vi "TCP Multiple Connections - Server.vi"() -> ()   [LabVIEW 2016]
doc: "该范例为支持客户端VI多个连接的TCP服务器VI。"
uses:
  controls/TCP Multiple Connections State.ctl
  controls/TCP Multiple Connections Data.ctl
panel:
  out "Boolean 3":bool
  out "flag":bool
  out "old":string
  in  "Boolean 2":bool
  in  "Boolean":bool
  out "值":cluster{"数值输入控件":dbl}
  out "错误输出":errorcluster
  out "temp":dbl format="%.2f"
  in  "loop":dbl
  out "sending msg":string
  out "data out":string
  in  "停止":bool
  out "连接数":i32
  # "概述：演示使用TCP函数初始化可向多个客户端VI发送数据的TCP服务器。\n操作步骤:\n1.运行VI。\n2.打开TCP Multiple Connections - Client 1.vi并按照前面板上的说明操作。\n3.打开TCP Multiple Connections - Client 2.vi并按照前面板上的说明操作。\n4.单击停止 停止VI运行。"
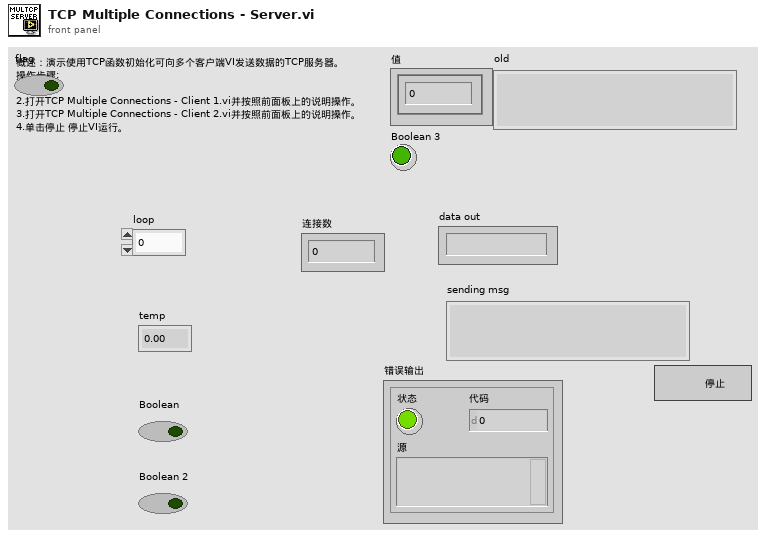
[diagram p1: front panel]
types:
  T1 = typedef "TCP Multiple Connections Data.ctl" = cluster{"客户端":refnum<k5>[], "侦听器":refnum<k5>}
  T2 = typedef "TCP Multiple Connections State.ctl" = enum16{"Initialize", "Status Check", "Send Data", "Stop"}
  T3 = enum16{"Standard", "Buffered", "CRLF", "Immediate"}
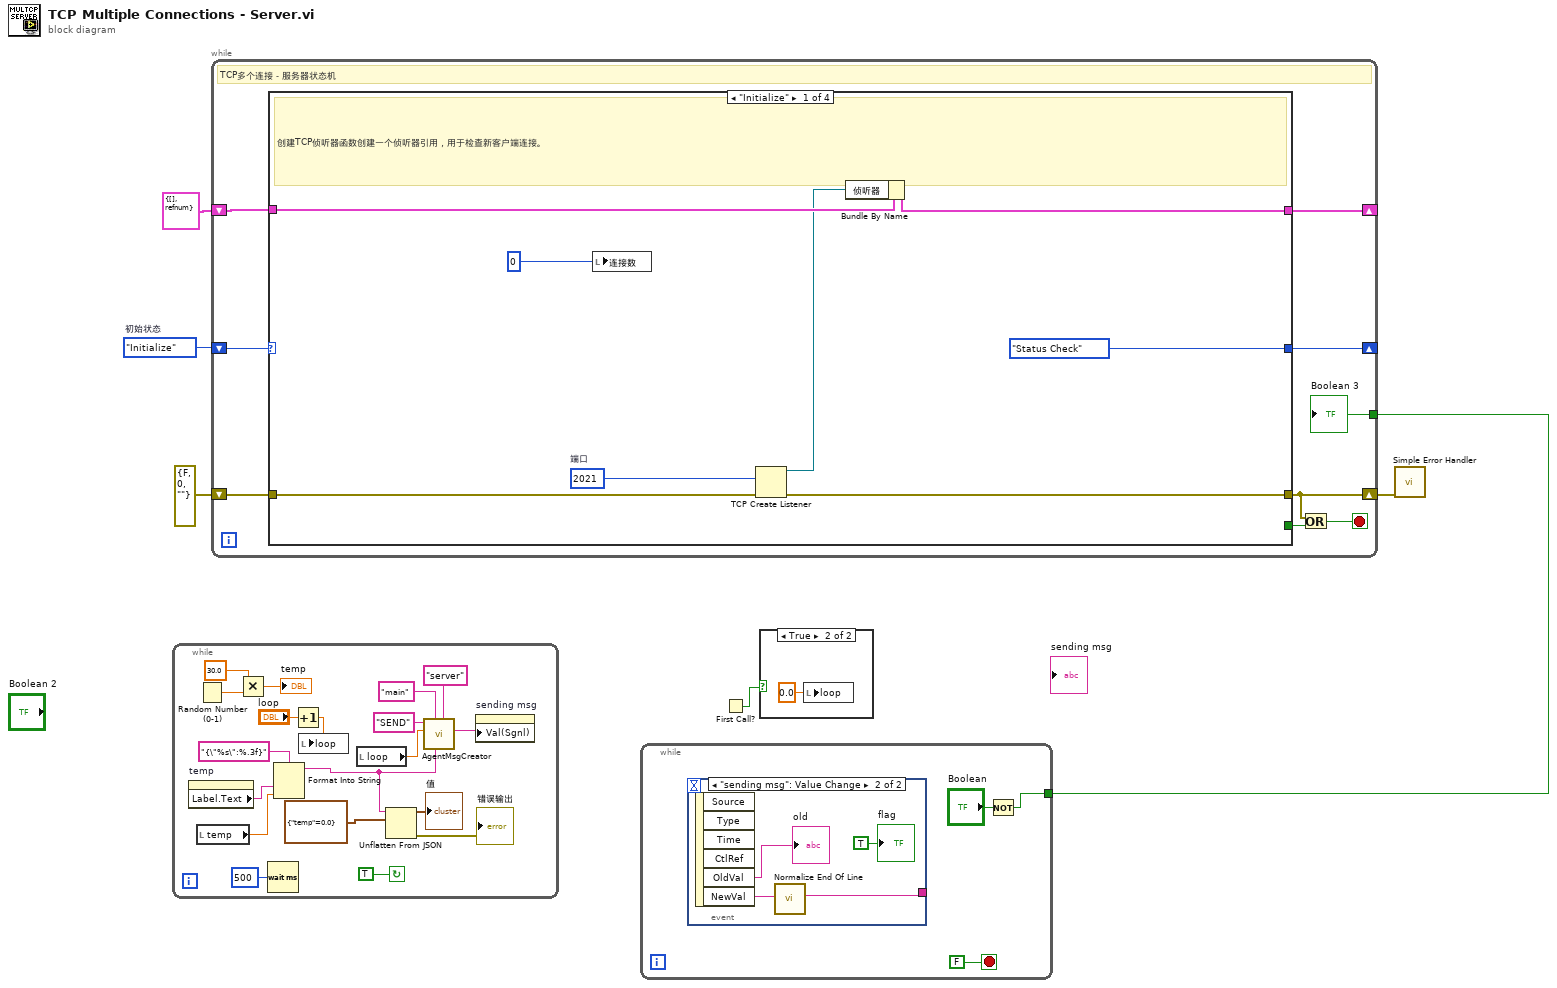
[diagram p0: block diagram]
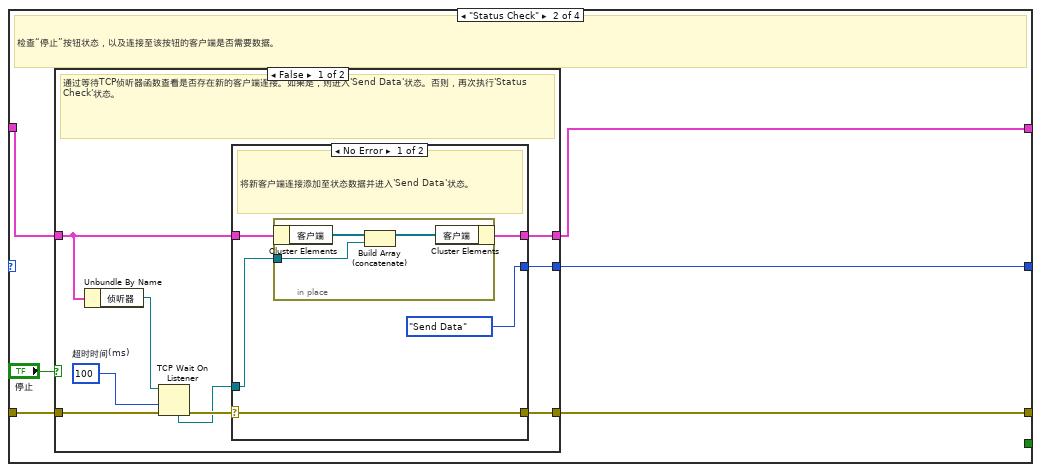
[diagram p2: hidden frame]
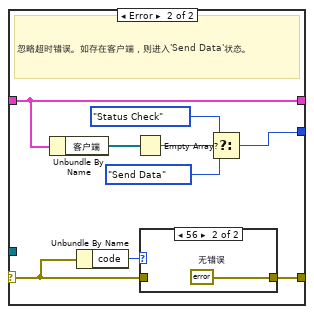
[diagram p3: hidden frame]
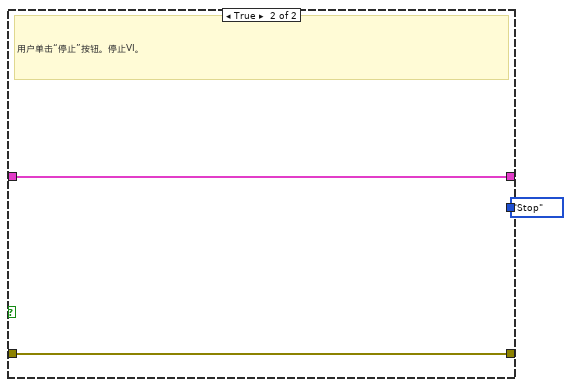
[diagram p5: hidden frame]
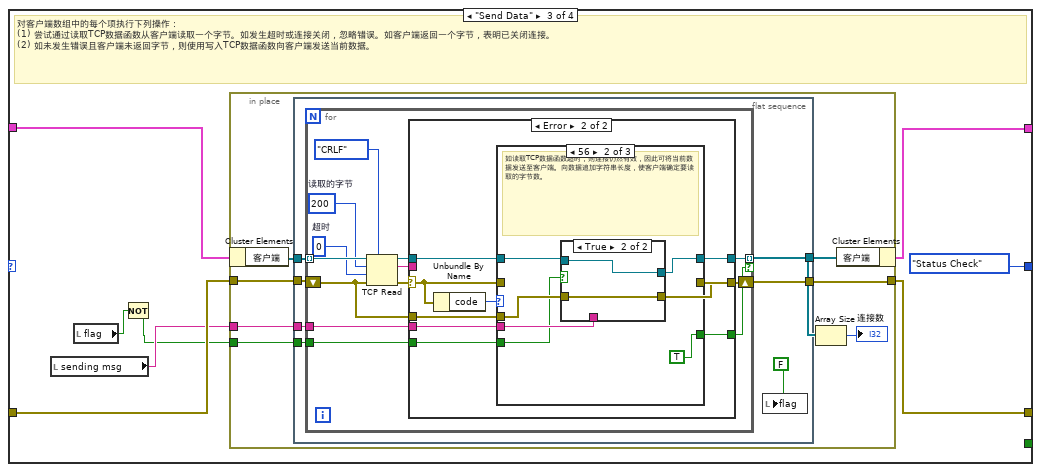
[diagram p6: hidden frame]
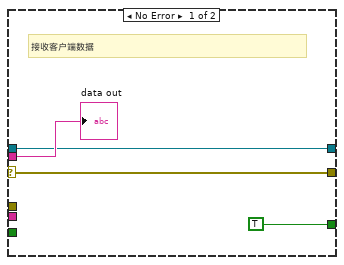
[diagram p7: hidden frame]
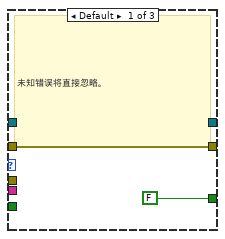
[diagram p8: hidden frame]
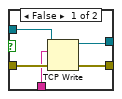
[diagram p9: hidden frame]
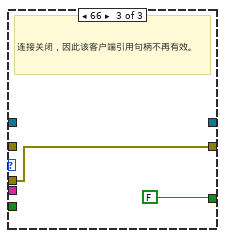
[diagram p10: hidden frame]
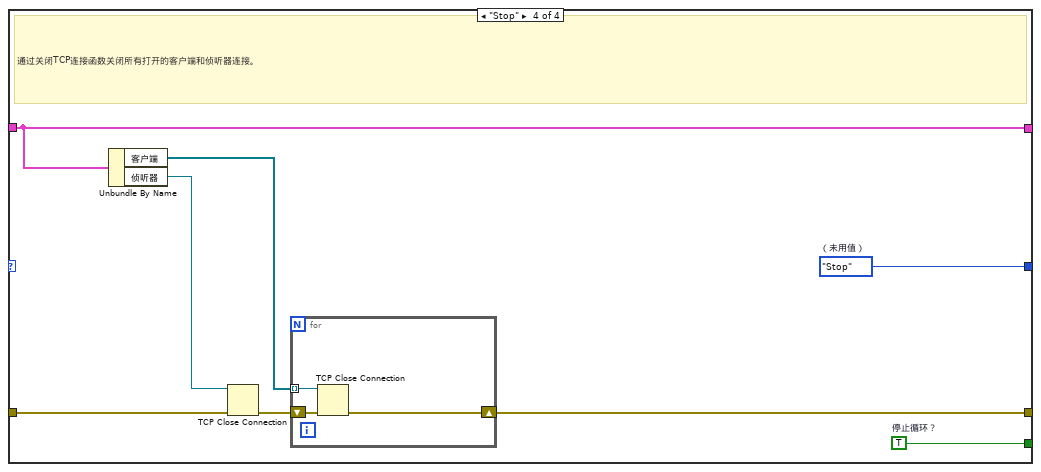
[diagram p11: hidden frame]
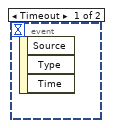
[diagram p12: hidden frame]
diagram:
  w2 = TCP_Multiple_Connections_State."Initialize"  # 初始状态
  n1 = while {
    stop <- TRUE continue-if-true
    n2 = property on="temp" class="DigNum (strict)"() -> ("Label.Text"=w15:string)  [unwired: 2 in, 2 out]
    n3 = Random Number (0-1)() -> (number: 0 to 1=w25:dbl)
    n4 = local read "temp"() -> (w14:dbl)
    n5 = Multiply(x=30.0, y=w25) -> (x*y=→"temp":dbl)
    n6 = Wait (ms)(milliseconds to wait=u32 500 ("等待时间（毫秒）")) -> ()  [unwired: 1 out]
    n7 = Format Into String(format string="{\"%s\":%.3f}" ("格式字符串"), w15, w14) -> (resulting string=w13:string)  [unwired: 2 in, 1 out]
    n8 = Increment(x="loop") -> (x+1=w7:dbl)
    n9 = local write "loop"(w7) -> ()
    n10 = local read "loop"() -> (w21:dbl)
    n11 = Unflatten From JSON(JSON string=w13, type and defaults=cluster{"temp":dbl} {"temp"=0.0}) -> (value=→"值":cluster{"temp":dbl}, error out=→"错误输出":errorcluster)  [unwired: 5 in]
    n12 = call "AgentMsgCreator.vi"("tp"="server", "dt"=w13, "id"="main", "rq"=w21, "cmd"="SEND") -> ("JSON字符串"=w9:string)  [unwired: 6 in]
    n13 = property on="sending msg" class="Str"("Val(Sgnl)"=w9) -> ()  [unwired: 2 in, 2 out]
  }
  n14 = while {
    tunnel: [w26] -> w1
    stop <- FALSE stop-if-true
    n15 = event shown="[1] \"sending msg\": Value Change" {
      selector: _ -> [_ _]
      dyn-events: _ -> [_ _]
      timeout: _ -> [_ _]
      tunnel: [_ w32] -> _
      event Timeout {
        n16 = event-data() -> ()  [unwired: 1 in, 3 out]
      }
      event "sending msg": Value Change {
        n17 = event-data() -> ("OldVal"=→"old":string, "NewVal"=w31:string)  [unwired: 1 in, 4 out]
        n18 = call <vilib>:"Normalize End Of Line.vi"("string in"=w31) -> ("string out"=w32:string)  [unwired: 7 in]
        "flag" <- TRUE ("flag")
      }
    }
    n19 = Not(x="Boolean") -> (.not. x?=w26:bool)
  }
  n20 = while {
    shift-right: [w40] -> _
    shift-left: w2 -> [w41]
    shift-right: [w38] -> _
    shift-left: T1 {"客户端"=[], "侦听器"=refnum} ("Data") -> [w39]
    shift-right: [w35] -> w5
    shift-left: errorcluster {"status"=FALSE, "code"=0, "source"=""} ("error constant") -> [w37]
    tunnel: w1 -> [w33]
    stop <- w34 stop-if-true
    # "TCP多个连接－服务器状态机"
    n21 = case shown="\"Initialize\"" w41 {
      tunnel: [TCP_Multiple_Connections_State."Status Check" ("States") w55 TCP_Multiple_Connections_State."Status Check" ("States") w153] -> w40
      tunnel: [_ _ _ w160] -> w36
      tunnel: w39 -> [w47 w51 w92 w159]
      tunnel: [w46 w50 w91 w159] -> w38
      tunnel: w37 -> [w49 w54 w94 w158]
      tunnel: [w48 w53 w93 w156] -> w35
      frame "Initialize" {
        w44 = u16 2021  # 端口
        # "创建TCP侦听器函数创建一个侦听器引用，用于检查新客户端连接。"
        n22 = local write "连接数"(0 ("Number of Client Connections")) -> ()
        n23 = TCP Create Listener(8:w49, 10:w44) -> (0:w48:errorcluster, 3:w45:refnum<k5>)  [unwired: 4 out]
        n24 = Bundle By Name(cluster=w47, "侦听器"=w45) -> (w46:T1)
      }
      frame "Status Check" {
        # "检查“停止”按钮状态，以及连接至该按钮的客户端是否需要数据。"
        n25 = case shown="False" "停止" {
          tunnel: [w64 TCP_Multiple_Connections_State."Stop" ("States")] -> w55
          tunnel: w54 -> [w63 w86]
          tunnel: [w56 w86] -> w53
          tunnel: w51 -> [w59 w85]
          tunnel: [w58 w85] -> w50
          frame False {
            w62 = 100  # 超时时间(ms)
            # "通过等待TCP侦听器函数查看是否存在新的客户端连接。如果是，则进入'Send Data'状态。否则，再次执行'Status Check'状态。"
            n26 = Unbundle By Name(w59) -> ("侦听器"=w57:refnum<k5>)
            n27 = TCP Wait On Listener(8:w63, 9:w62, 11:w57) -> (0:w61:errorcluster, 4:w60:refnum<k5>)  [unwired: 4 out]
            n28 = case shown="No Error" w61 {
              selector: w61 -> [w67 w81]
              tunnel: [TCP_Multiple_Connections_State."Send Data" ("States") w75] -> w64
              tunnel: w60 -> [w68 _]
              tunnel: w59 -> [w69 w78]
              tunnel: [w66 w78] -> w58
              tunnel: [w67 w79] -> w56
              frame No Error {
                # "将新客户端连接添加至状态数据并进入'Send Data'状态。"
                n29 = in-place {
                  in-place-border: w68 -> [w70]
                  n30 = in-place-cluster #1(w69) -> ("客户端"=w72:refnum<k5>[])
                  n31 = Build Array (concatenate)(w72, w70) -> (w71:refnum<k5>[])
                  n32 = in-place-cluster #1("客户端"=w71) -> (w66:T1)
                }
              }
              frame Error {
                # "忽略超时错误。如存在客户端，则进入'Send Data'状态。"
                n33 = Unbundle By Name(w78) -> ("客户端"=w77:refnum<k5>[])
                n34 = Unbundle By Name(w81) -> ("code"=w80:i32)
                n35 = Empty Array?(array=w77) -> (empty?=w76:bool)
                n36 = case shown="56" w80 {
                  tunnel: w81 -> [w82 _]
                  tunnel: [w82 w83] -> w79
                  frame Default {
                  }
                  frame 56 {
                    w83 = errorcluster {"status"=FALSE, "code"=0, "source"=""}  # 无错误
                  }
                }
                n37 = Select(t=TCP_Multiple_Connections_State."Status Check" ("States"), s=w76, f=TCP_Multiple_Connections_State."Send Data" ("States")) -> (s? t:f=w75:T2)
              }
            }
          }
          frame True {
            # "用户单击“停止”按钮。停止VI。"
          }
        }
      }
      frame "Send Data" {
        # "对客户端数组中的每个项执行下列操作：\n(1) 尝试通过读取TCP数据函数从客户端读取一个字节。如发生超时或连接关闭，忽略错误。如客户端返回一个字节，表明已关闭连接。\n(2) 如未发生错误且客户端未返回字节，则使用写入TCP数据函数向客户端发送当前数据。"
        n38 = local read "sending msg"() -> (w89:string)
        n39 = local read "flag"() -> (w87:bool)
        n40 = Not(x=w87) -> (.not. x?=w88:bool)
        n41 = in-place {
          in-place-border: w94 -> [w101]
          in-place-border: [w100] -> w93
          in-place-border: w89 -> [w96]
          in-place-border: w88 -> [w95]
          n42 = in-place-cluster #2(w92) -> ("客户端"=w98:refnum<k5>[])
          n43 = flat-sequence {
            tunnel: w101 -> [w108]
            tunnel: [w107] -> w100
            tunnel: w98 -> [w106]
            tunnel: [w105] -> w97
            tunnel: w96 -> [w104]
            tunnel: w95 -> [w103]
            frame #0 {
              n44 = for {
                tunnel: w106 -> [w121] mode=indexing
                shift-right: [w113] -> w107
                shift-left: w108 -> [w112]
                tunnel: [w115] -> w105 mode=indexing if=w114
                tunnel: w104 -> [w110]
                tunnel: w103 -> [w109]
                w118 = 0  # 超时
                w119 = 200  # 读取的字节
                n45 = TCP Read(connection ID=w121, bytes to read=w119, error in (no error)=w112, 7:T3."CRLF" ("模式（标准）"), 9:w118) -> (connection ID out=w120:refnum<k5>, data out=w116:string, error out=w117:errorcluster)
                n46 = case shown="Error" w117 {
                  selector: w117 -> [w124 w133]
                  tunnel: w120 -> [w122 w130]
                  tunnel: w116 -> [w123 _]
                  tunnel: [w122 w128] -> w115
                  tunnel: [TRUE w129] -> w114
                  tunnel: [w124 w132] -> w113
                  tunnel: w112 -> [_ w131]
                  tunnel: w110 -> [_ w127]
                  tunnel: w109 -> [_ w126]
                  frame No Error {
                    # "接收客户端数据"
                    # "如客户端发送了数据，则通知应关闭连接。"
                    "data out" <- w123
                  }
                  frame Error {
                    # "忽略连接关闭和超时错误"
                    n47 = Unbundle By Name(w133) -> ("code"=w134:i32)
                    n48 = case shown="56" w134 {
                      tunnel: w133 -> [w136 _ _]
                      tunnel: [w136 w143 w152] -> w132
                      tunnel: w131 -> [_ w139 w152]
                      tunnel: w130 -> [_ w142 _]
                      tunnel: [FALSE TRUE FALSE] -> w129
                      tunnel: [_ w141 _] -> w128
                      tunnel: w127 -> [_ w138 _]
                      tunnel: w126 -> [_ w137 _]
                      frame Default {
                        # "未知错误将直接忽略。"
                      }
                      frame 56 {
                        # "如读取TCP数据函数超时，则连接仍然有效，因此可将当前数据发送至客户端。向数据追加字符串长度，使客户端确定要读取的字节数。"
                        n49 = case shown="True" w137 {
                          tunnel: [w144 w150] -> w143
                          tunnel: w142 -> [w148 w149]
                          tunnel: [w145 w149] -> w141
                          tunnel: w139 -> [w147 w150]
                          tunnel: w138 -> [w146 _]
                          frame False {
                            n50 = TCP Write(connection ID=w148, data in=w146, error in (no error)=w147) -> (connection ID out=w145:refnum<k5>, error out=w144:errorcluster)  [unwired: 2 out]
                          }
                          frame True {
                          }
                        }
                      }
                      frame 66 {
                        # "连接关闭，因此该客户端引用句柄不再有效。"
                      }
                    }
                  }
                }
              }
              n51 = local write "flag"(FALSE ("flag")) -> ()
            }
          }
          n52 = Array Size(array=w97) -> (size(s)=→"连接数":i32)
          n53 = in-place-cluster #2("客户端"=w97) -> (w91:T1)
        }
      }
      frame "Stop" {
        w153 = TCP_Multiple_Connections_State."Stop"  # （未用值）
        w160 = TRUE  # 停止循环？
        # "通过关闭TCP连接函数关闭所有打开的客户端和侦听器连接。"
        n54 = Unbundle By Name(w159) -> ("客户端"=w157:refnum<k5>[], "侦听器"=w154:refnum<k5>)
        n55 = TCP Close Connection(connection ID=w154, error in (no error)=w158) -> (error out=w155:errorcluster)  [unwired: 1 in, 1 out]
        n56 = for {
          shift-right: [w162] -> w156
          shift-left: w155 -> [w163]
          tunnel: w157 -> [w161] mode=indexing
          n57 = TCP Close Connection(connection ID=w161, error in (no error)=w163) -> (error out=w162:errorcluster)  [unwired: 1 in, 1 out]
        }
      }
    }
    n58 = Or(x=w35, y=w36) -> (x .or. y?=w34:bool)
    "Boolean 3" <- w33
  }
  n59 = First Call?() -> (First Call?: T/F=w6:bool)
  n60 = case shown="True" w6 {
    frame False {
    }
    frame True {
      n61 = local write "loop"(0.0 ("数值")) -> ()
    }
  }
  n62 = call <vilib>:"Simple Error Handler.vi"("error in (no error)"=w5) -> ()  [unwired: 4 in, 5 out]
